vi "Maui.Config.Locate.vi"(6 "Create?":bool, 8 "error in (no error)":errorcluster, 9 "Path":path, 10 "Application Name":string, 11 "Maui.Config in":refnum<class "Maui.Config.lvclass">) -> (0 "error out":errorcluster, 1 "Exists?":bool, 2 "Path":path, 3 "Maui.Config out":refnum<class "Maui.Config.lvclass">, 4 "Created?":bool)   [LabVIEW 2020, in "Maui.Config.lvclass"]
uses:
  Maui.Config.lvclass
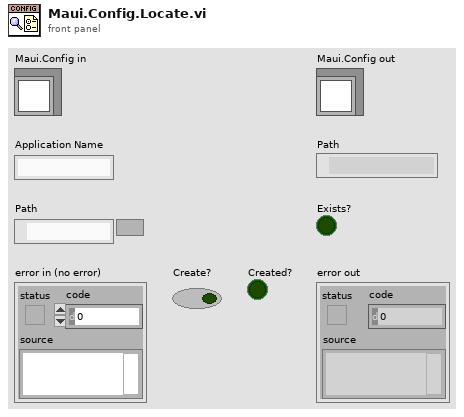
[diagram p1: front panel]
types:
  T1 = enum16{"open", "replace", "create", "open or create", "replace or create", "replace or create with confirmation"}
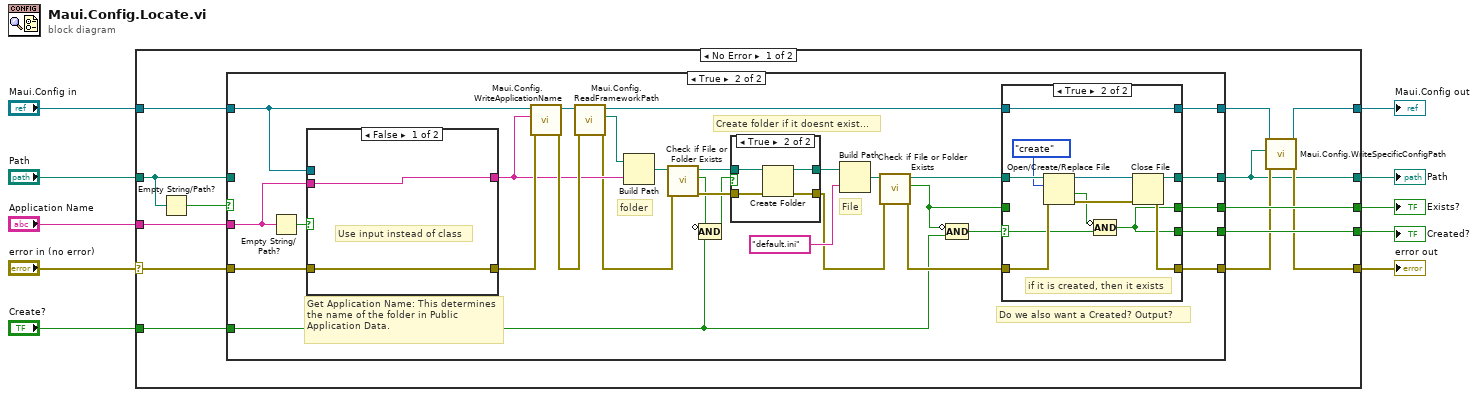
[diagram p0: block diagram]
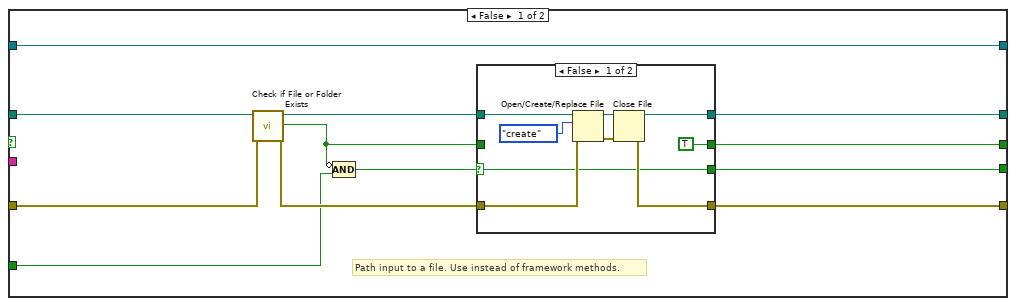
[diagram p2: hidden frame]
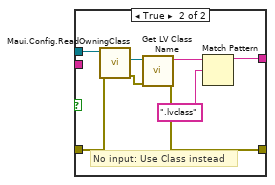
[diagram p6: hidden frame]
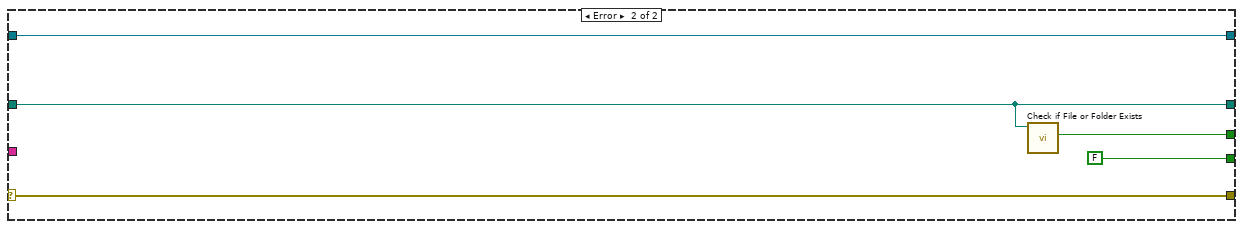
[diagram p7: hidden frame]
diagram:
  n1 = case shown="No Error" "error in (no error)" {
    selector: "error in (no error)" -> [w23 w113]
    tunnel: [w13 w113] -> w9
    tunnel: [w15 w115] -> w7
    tunnel: "Maui.Config in" -> [w21 w115]
    tunnel: "Application Name" -> [w22 _]
    tunnel: "Path" -> [w11 w112]
    tunnel: "Create?" -> [w19 _]
    tunnel: [w18 w111] -> w3
    tunnel: [w17 FALSE] -> w2
    tunnel: [w12 w112] -> w1
    frame No Error {
      n2 = Empty String/Path?(string/path=w11) -> (empty?=w20:bool)
      n3 = case shown="True" w20 {
        tunnel: w22 -> [_ w73]
        tunnel: [w35 w67] -> w16
        tunnel: w21 -> [w35 w71]
        tunnel: [w32 w76] -> w14
        tunnel: w23 -> [w33 w77]
        tunnel: w19 -> [w27 w49]
        tunnel: [w29 w60] -> w12
        tunnel: [w26 w59] -> w18
        tunnel: [w24 w58] -> w17
        tunnel: w11 -> [w34 _]
        frame False {
          # "Path input to a file. Use instead of framework methods."
          n4 = call <vilib>:"Check if File or Folder Exists.vi"("error in (no error)"=w33, "path"=w34) -> ("error out"=w31:errorcluster, "file or folder exists?"=w25:bool, "dup path"=w30:path)  [unwired: 7 in]
          n5 = Compound Arithmetic op=AND(invert w25, w27) -> (w28:bool)
          n6 = case shown="False" w28 {
            selector: w28 -> [w36 w45]
            tunnel: [w38 w48] -> w32
            tunnel: w31 -> [w41 w48]
            tunnel: w30 -> [w39 w47]
            tunnel: [w40 w47] -> w29
            tunnel: [TRUE w46] -> w26
            tunnel: w25 -> [_ w46]
            tunnel: [w36 w45] -> w24
            frame False {
              n7 = Open/Create/Replace File(file path (use dialog)=w39, error in=w41, operation (0:open)=T1."create") -> (refnum out=w43:refnum<file>, error out=w42:errorcluster)  [unwired: 3 in, 1 out]
              n8 = Close File(refnum=w43, error in=w42) -> (path=w40:path, error out=w38:errorcluster)
            }
            frame True {
            }
          }
        }
        frame True {
          # "Create folder if it doesnt exist..."
          # "Do we also want a Created? Output?"
          # "File"
          # "Get Application Name: This determines the name of the folder in Public Application Data."
          # "folder"
          n9 = Empty String/Path?(string/path=w73) -> (empty?=w72:bool)
          n10 = case shown="False" w72 {
            tunnel: w71 -> [_ w107]
            tunnel: w77 -> [w102 w109]
            tunnel: [w101 w103] -> w68
            tunnel: w73 -> [w101 _]
            tunnel: [w102 w108] -> w78
            frame False {
              # "Use input instead of class"
            }
            frame True {
              # "No input: Use Class instead"
              n11 = call "Maui.Config.ReadOwningClass.vi"("error in (no error)"=w109, "Maui.Config in"=w107) -> ("error out"=w110:errorcluster, "Owning Class"=w106:refnum<class>)  [unwired: 7 in, 1 out]
              n12 = call <vilib>:"Get LV Class Name.vi"("error in (no error)"=w110, "object"=w106) -> ("error out"=w108:errorcluster, "class name"=w105:string)  [unwired: 8 in]
              n13 = Match Pattern(string=w105, regular expression=".lvclass") -> (before substring=w103:string)  [unwired: 1 in, 3 out]
            }
          }
          n14 = call "Maui.Config.WriteApplicationName.vi"("error in (no error)"=w78, "Application Name"=w68, "Maui.Config in"=w71) -> ("error out"=w74:errorcluster, "Maui.Config out"=w70:refnum<class "Maui.Config.lvclass">)  [unwired: 7 in]
          n15 = call "Maui.Config.ReadFrameworkPath.vi"("error in (no error)"=w74, "Maui.Config in"=w70) -> ("error out"=w54:errorcluster, "Framework Path"=w69:path, "Maui.Config out"=w66:refnum<class "Maui.Config.lvclass">)  [unwired: 7 in]
          n16 = Build Path(base path=w69, name or relative path=w68) -> (appended path=w57:path)
          n17 = call <vilib>:"Check if File or Folder Exists.vi"("error in (no error)"=w54, "path"=w57) -> ("error out"=w55:errorcluster, "file or folder exists?"=w51:bool, "dup path"=w56:path)  [unwired: 7 in]
          n18 = Compound Arithmetic op=AND(invert w51, w49) -> (w50:bool)
          n19 = case shown="True" w50 {
            tunnel: w56 -> [w80 w84]
            tunnel: w55 -> [w79 w83]
            tunnel: [w79 w82] -> w53
            tunnel: [w80 w81] -> w52
            frame False {
            }
            frame True {
              n20 = Create Folder(path (use dialog)=w84, error in=w83) -> (created path=w81:path, error out=w82:errorcluster)  [unwired: 1 in, 1 out]
            }
          }
          n21 = Build Path(base path=w52, name or relative path="default.ini") -> (appended path=w61:path)
          n22 = call <vilib>:"Check if File or Folder Exists.vi"("error in (no error)"=w53, "path"=w61) -> ("error out"=w75:errorcluster, "file or folder exists?"=w63:bool, "dup path"=w65:path)  [unwired: 7 in]
          n23 = Compound Arithmetic op=AND(invert w63, w49) -> (w64:bool)
          n24 = case shown="True" w64 {
            selector: w64 -> [w85 w91]
            tunnel: [w88 w100] -> w67
            tunnel: w66 -> [w88 w100]
            tunnel: [w89 w94] -> w76
            tunnel: w75 -> [w89 w95]
            tunnel: w65 -> [w86 w99]
            tunnel: w63 -> [w87 _]
            tunnel: [w86 w93] -> w60
            tunnel: [w87 w90] -> w59
            tunnel: [w85 w90] -> w58
            frame False {
            }
            frame True {
              # "if it is created, then it exists"
              n25 = Open/Create/Replace File(file path (use dialog)=w99, error in=w95, operation (0:open)=T1."create") -> (refnum out=w97:refnum<file>, cancelled=w92:bool, error out=w96:errorcluster)  [unwired: 3 in]
              n26 = Compound Arithmetic op=AND(invert w92, w91) -> (w90:bool)
              n27 = Close File(refnum=w97, error in=w96) -> (path=w93:path, error out=w94:errorcluster)
            }
          }
        }
      }
      n28 = call "Maui.Config.WriteSpecificConfigPath.vi"("error in (no error)"=w14, "Specific Configuration"=w12, "Maui.Config in"=w16) -> ("error out"=w13:errorcluster, "Maui.Config out"=w15:refnum<class "Maui.Config.lvclass">)  [unwired: 7 in]
    }
    frame Error {
      n29 = call <vilib>:"Check if File or Folder Exists.vi"("path"=w112) -> ("file or folder exists?"=w111:bool)  [unwired: 8 in, 2 out]
    }
  }
  "error out" <- w9
  "Maui.Config out" <- w7
  "Exists?" <- w3
  "Created?" <- w2
  "Path" <- w1
